vi "GetTimerResetCondition.vi"(3 "error in (no error)":errorcluster, 4 "Reset Timer Condition":u8(ring) items=["External Trigger In", "External Modulation In", "Wait Exit", "Conditional jump", "Dynamic Jump"], 5 "VISA resource name":refnum<visa-resource-name>) -> (0 "error out":errorcluster, 1 "Ext Mod State":bool, 2 "VISA resource name out":refnum<visa-resource-name>)   [LabVIEW 2020, in "Active Technologies AWG3000.lvlib"]
uses:
  Active Technologies AWG3000.lvlib
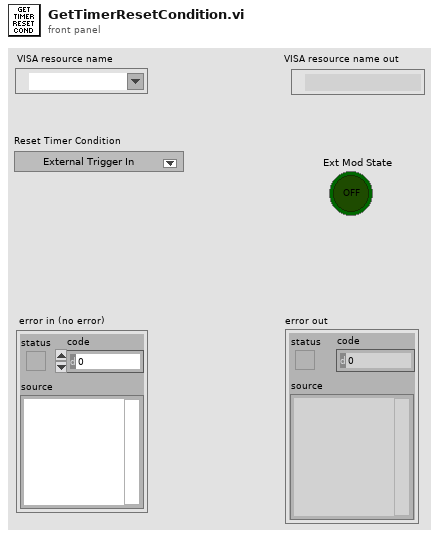
[diagram p1: front panel]
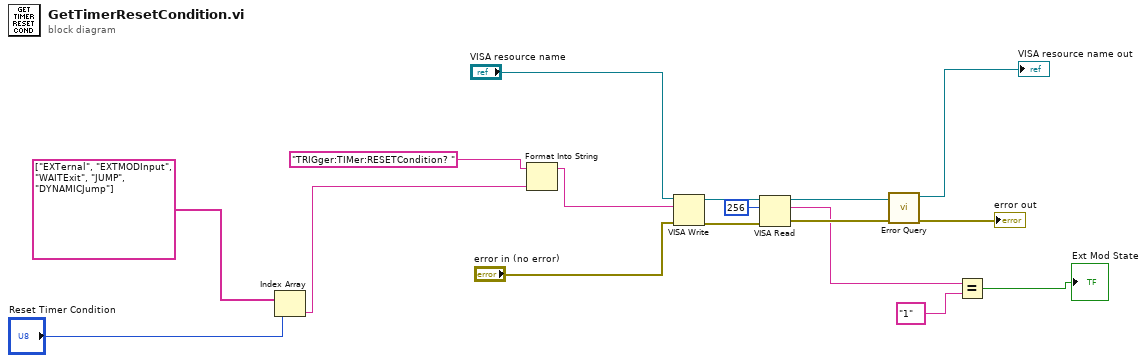
[diagram p0: block diagram]
diagram:
  n1 = Index Array(array=string[] ["EXTernal", "EXTMODInput", "WAITExit", "JUMP", "DYNAMICJump"], index="Reset Timer Condition") -> (element=w4:string)
  n2 = Format Into String(initial string="TRIGger:TIMer:RESETCondition? " ("write buffer"), w4) -> (resulting string=w1:string)  [unwired: 2 in, 1 out]
  n3 = VISA Write(VISA resource name="VISA resource name", write buffer=w1, error in (no error)="error in (no error)") -> (VISA resource name out=w15:refnum<visa-resource-name>, error out=w14:errorcluster)  [unwired: 1 out]
  n4 = VISA Read(VISA resource name=w15, byte count=u32 256, error in (no error)=w14) -> (VISA resource name out=w12:refnum<visa-resource-name>, read buffer=w8:string, error out=w11:errorcluster)  [unwired: 1 out]
  n5 = call "Error Query.vi"("error in (no error)"=w11, "VISA resource name"=w12) -> ("error out"=→"error out":errorcluster, "VISA resource name out"=→"VISA resource name out":refnum<visa-resource-name>)  [unwired: 6 in, 2 out]
  n6 = Equal?(x=w8, y="1") -> (x = y?=→"Ext Mod State":bool)
